vi "Constant - Timeout (ms).vi"() -> (3 "timeout (ms)":i32=3000)   [LabVIEW 2020]
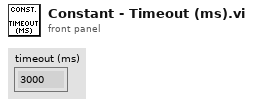
[diagram p1: front panel]
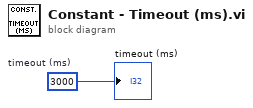
[diagram p0: block diagram]
diagram:
  w1 = 3000  # timeout (ms)
  "timeout (ms)" <- w1
